vi "Untitled 3.vi"() -> ()   [LabVIEW 2019]
uses:
  <vilib>/sound2/lvsound2.llb/Sound Data Format.ctl
  <vilib>/sound2/lvsound2.llb/Sampling Mode.ctl
  <vilib>/Analysis/4window.llb/Gaussian Window (DBL).vi
  <vilib>/sound2/lvsound2.llb/Sound Output Write (DBL Single).vi
  <vilib>/Analysis/NI_AALBase.lvlib
  <vilib>/Analysis/NI_AALPro.lvlib
panel:
  in  "standard deviation":dbl=0.2
  out "Waveform Graph 2":dbl[](graph)
  in  "sine wave freq":dbl=0.0078125 format="%0.4e"
  in  "chirp/gaussian":bool
  in  "number of periods":i32
  in  "f1":dbl
  in  "f2":dbl
  in  "amplitude":dbl=1.0 format="%0.2f"
  out "Waveform Graph":dbl[](graph)
  in  "time (secs)":dbl
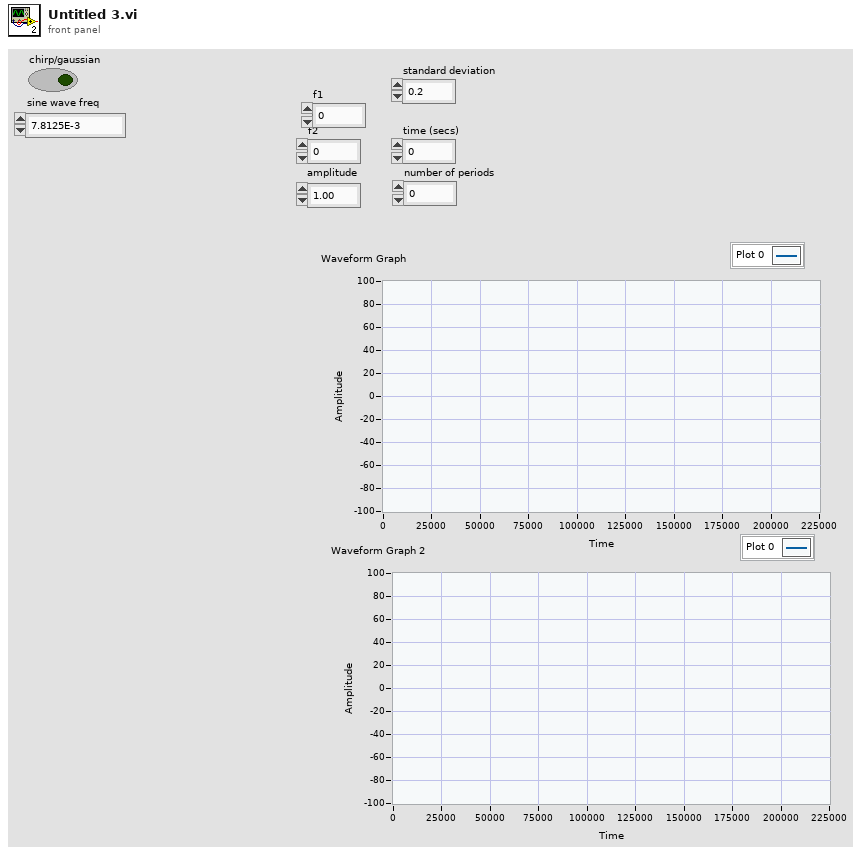
[diagram p1: front panel]
types:
  T1 = typedef "Sampling Mode.ctl" = i32
  T2 = typedef "Sound Data Format.ctl" = cluster{"sample rate (S/s)":dbl, "number of channels":i32, "bits per sample":i32}
  T3 = typedef "Sound Output Task ID.ctl" = u32
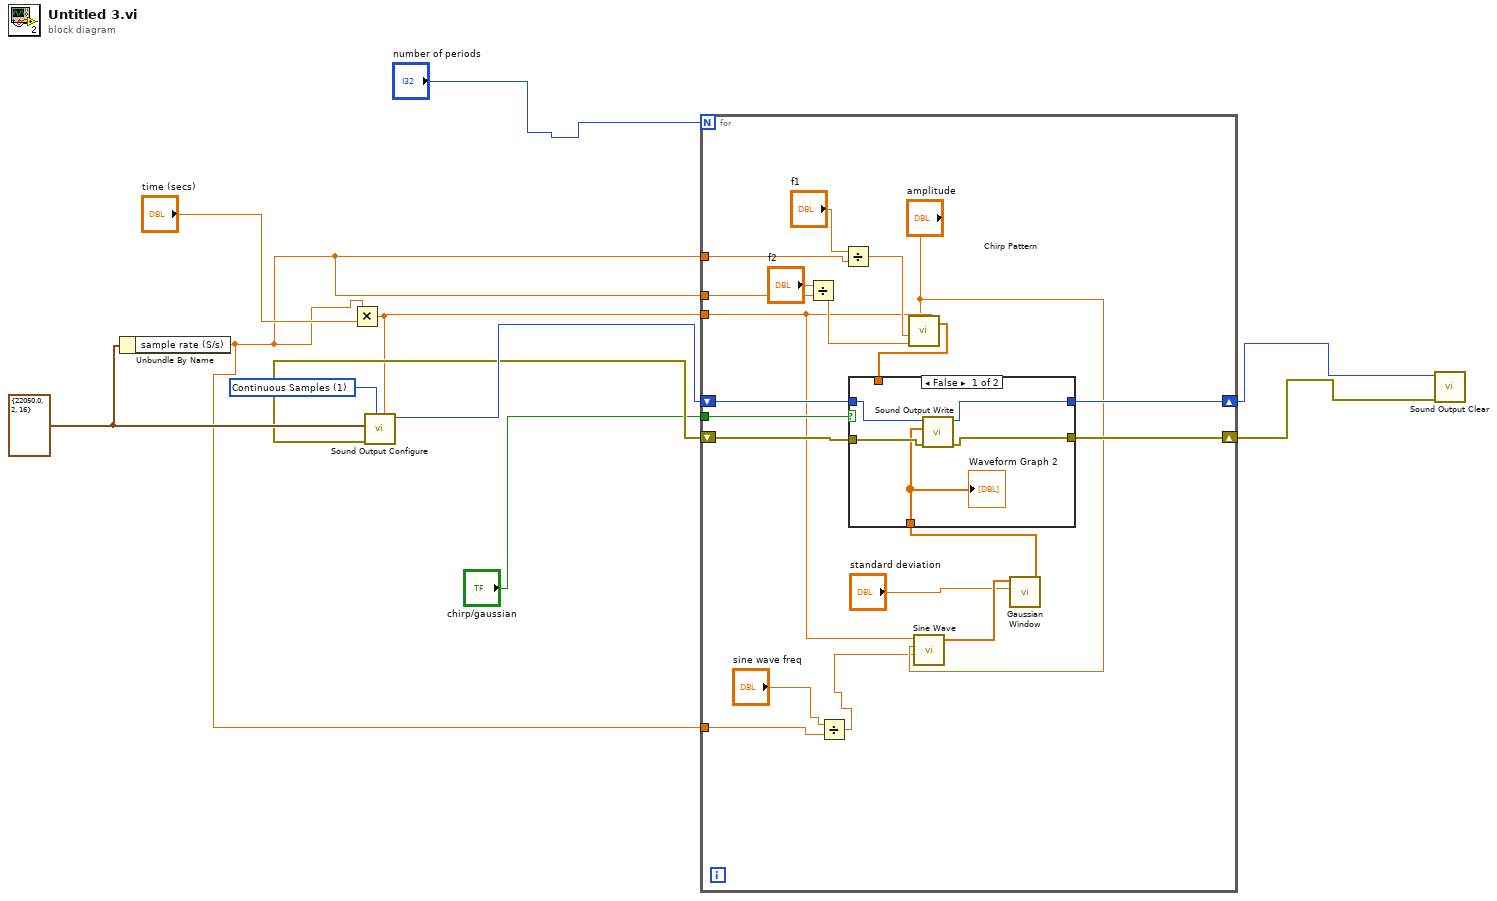
[diagram p0: block diagram]
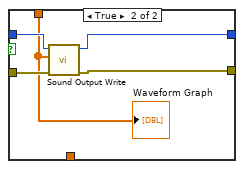
[diagram p2: hidden frame]
diagram:
  w10 = T1 1 items=["Finite Samples", "Continuous Samples"] ("sample mode")
  w11 = T2 {"sample rate (S/s)"=22050.0, "number of channels"=2, "bits per sample"=16} ("sound format")
  n1 = Unbundle By Name(w11) -> ("sample rate (S/s)"=w1:dbl)
  n2 = Multiply(x=w1, y="time (secs)") -> (x*y=w4:dbl)
  n3 = call <vilib>:"Sound Output Configure.vi"("number of samples/ch"=w4, "sample mode"=w10, "sound format"=w11) -> ("error out"=w7:errorcluster, "task ID"=w8:T3)  [unwired: 7 in]
  n4 = for {
    N: "number of periods" -> [_]
    tunnel: w4 -> [w19]
    tunnel: w1 -> [w27]
    tunnel: w1 -> [w23]
    shift-right: [w30] -> w5
    shift-left: w7 -> [w31]
    shift-right: [w28] -> w6
    shift-left: w8 -> [w29]
    tunnel: "chirp/gaussian" -> [w20]
    tunnel: w1 -> [w15]
    n5 = Divide(x="f2", y=w23) -> (x/y=w24:dbl)
    n6 = Divide(x="sine wave freq", y=w15) -> (x/y=w17:dbl)
    n7 = Divide(x="f1", y=w27) -> (x/y=w26:dbl)
    n8 = call <vilib>:"Chirp Pattern.vi"("f2"=w24, "f1"=w26, "amplitude"="amplitude", "samples"=w19) -> ("Chirp Pattern"=w21:dbl[])  [unwired: 1 out]
    n9 = call <vilib>:"Sine Wave.vi"("samples"=w19, "amplitude"="amplitude", "frequency"=w17) -> ("sine wave"=w14:dbl[])  [unwired: 2 in, 2 out]
    n10 = call-poly <vilib>:"Gaussian Window.vi"("standard deviation"="standard deviation", "X"=w14) -> ("Windowed X"=w13:dbl[])  [unwired: 8 in, 1 out]
    n11 = case shown="False" w20 {
      tunnel: w31 -> [w35 w41]
      tunnel: [w34 w40] -> w30
      tunnel: w29 -> [w36 w39]
      tunnel: [w33 w38] -> w28
      tunnel: w21 -> [_ w37]
      tunnel: w13 -> [w32 _]
      frame False {
        n12 = call-poly <vilib>:"Sound Output Write.vi"("error in (no error)"=w35, "data"=w32, "task ID"=w36) -> ("error out"=w34:errorcluster, "task ID out"=w33:T3)  [unwired: 7 in]
        "Waveform Graph 2" <- w32
      }
      frame True {
        n13 = call-poly <vilib>:"Sound Output Write.vi"("error in (no error)"=w41, "data"=w37, "task ID"=w39) -> ("error out"=w40:errorcluster, "task ID out"=w38:T3)  [unwired: 7 in]
        "Waveform Graph" <- w37
      }
    }
  }
  n14 = call <vilib>:"Sound Output Clear.vi"("error in (no error)"=w5, "task ID"=w6) -> ()  [unwired: 9 in, 1 out]
